vi "用探测器信息 初始化 探头属性.vi"(11 "探测器信息":T1) -> (3 "探头属性":T4)   [LabVIEW 2017]
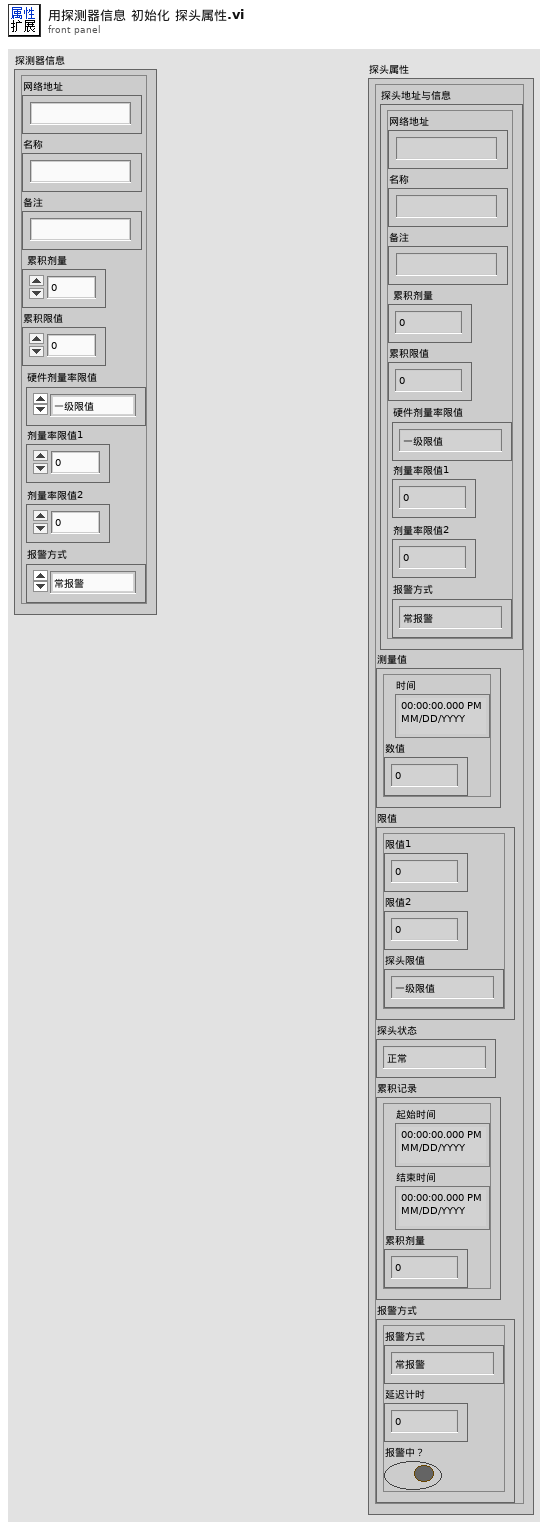
[diagram p1: front panel]
types:
  T1 = typedef "探测器信息.ctl" = cluster{"网络地址":string, "名称":string, "备注":string, "累积剂量":dbl, "累积限值":dbl, "硬件剂量率限值":T2, "剂量率限值1":dbl, "剂量率限值2":dbl, "报警方式":T3}
  T2 = typedef "探头剂量率限值选择.ctl" = enum16{"一级限值", "二级限值"}
  T3 = typedef "报警方式选择.ctl" = enum16{"常报警", "自动静音", "手动静音"}
  T4 = typedef "探头属性.ctl" = cluster{"探头地址与信息":T1, "测量值":T5, "限值":T6, "探头状态":T7, "累积记录":T8, "报警方式":T9}
  T5 = typedef "测量值.ctl" = cluster{"时间":timestamp, "数值":dbl}
  T6 = typedef "剂量率限值.ctl" = cluster{"限值1":dbl, "限值2":dbl, "探头限值":T2}
  T7 = typedef "探头状态.ctl" = enum16{"正常", "离线", "禁用", "一级报警", "二级报警", "累积报警"}
  T8 = typedef "单条累积记录.ctl" = cluster{"起始时间":timestamp, "结束时间":timestamp, "累积剂量":dbl}
  T9 = typedef "报警方式.ctl" = cluster{"报警方式":T3, "延迟计时":u16, "报警中？":bool}
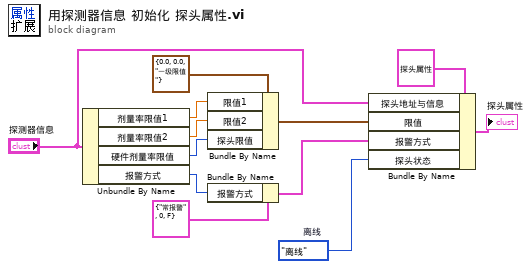
[diagram p0: block diagram]
diagram:
  w1 = 探头状态."离线"  # 离线
  n1 = Unbundle By Name("探测器信息") -> ("剂量率限值1"=w6:dbl, "剂量率限值2"=w5:dbl, "硬件剂量率限值"=w4:T2, "报警方式"=w3:T3)
  n2 = Bundle By Name(cluster=T6 {"限值1"=0.0, "限值2"=0.0, "探头限值"=enum."一级限值"} ("限值"), "限值1"=w6, "限值2"=w5, "探头限值"=w4) -> (w9:T6)
  n3 = Bundle By Name(cluster=T9 {"报警方式"=enum."常报警", "延迟计时"=0, "报警中？"=FALSE} ("报警方式"), "报警方式"=w3) -> (w7:T9)
  n4 = Bundle By Name(cluster=T4 {"探头地址与信息"={"网络地址"="", "名称"="", "备注"="", "累积剂量"=0.0, "累积限值"=0.0, "硬件剂量率限值"=enum."一级限值", "剂量率限值1"=0.0, "剂量率限值2"=0.0, "报警方式"=enum."常报警"}, "测量值"={"时间"=timestamp(0 s since 1904-01-01), "数值"=0.0}, "限值"={"限值1"=0.0, "限值2"=0.0, "探头限值"=enum."一级限值"}, "探头状态"=enum."正常", "累积记录"={"起始时间"=timestamp(0 s since 1904-01-01), "结束时间"=timestamp(0 s since 1904-01-01), "累积剂量"=0.0}, "报警方式"={"报警方式"=enum."常报警", "延迟计时"=0, "报警中？"=FALSE}} ("探头属性"), "探头地址与信息"="探测器信息", "限值"=w9, "报警方式"=w7, "探头状态"=w1) -> (→"探头属性":T4)
